vi "Get Control Indexes.vi"(10 "data allocations":T2, 11 "Sequencer Module configuration in":refnum<class "Sequencer Module configuration.lvclass">) -> (0 "error out":errorcluster, 2 "Sequencer Control Index":T1)   [LabVIEW 2015, in "Sequencer Module runtime.lvclass"]
uses:
  Sequencer Module runtime.lvclass
  <vilib>/NI/Tag Bus Module Framework/channel/data tables.ctl
  <vilib>/NI/Tag Bus/dictionary/data dictionary.lvclass
  <vilib>/NI/Tag Bus/dictionary table pair.ctl
  <vilib>/NI/Tag Bus/table/data table.ctl
  configuration/Sequencer Module configuration.lvclass
  Sequencer Control Index.ctl
  <vilib>/NI/Tag Bus Module Framework/channel/TBM channel.lvclass/TBM channel.ctl
  <vilib>/NI/Tag Bus/tag/tag descriptor.lvclass/tag descriptor.ctl
  <vilib>/NI/Tag Bus/tag/read tag name.vi
  <vilib>/NI/Tag Bus/tag/read data type.vi
  <vilib>/NI/Tag Bus/dictionary/locate tag.vi
  <vilib>/NI/Tag Bus Module Framework/channel/TBM channel.lvclass
  <vilib>/NI/Tag Bus/table/data table.lvlib
  <vilib>/NI/Tag Bus/tag bus.lvlib
types:
  T1 = typedef "Sequencer Module runtime.lvclass/Sequencer Control Index.ctl" = cluster{"Start":i32, "Change Sequence":i32, "New Sequence":i32, "Pause":i32}
  T2 = typedef "TBM channel.lvclass/data tables.ctl" = cluster{"input data":T3, "processing parameter":T3, "processing result":T3, "output data":T3}
  T3 = typedef "tag bus.lvlib/dictionary table pair.ctl" = cluster{"data dictionary":refnum<class "data dictionary.lvclass">, "data table":T4}
  T4 = typedef "tag bus.lvlib/data table.lvlib/data table.ctl" = cluster{"Double":dbl[], "Single":sgl[], "I64":i64[], "I32":i32[], "I16":i16[], "I8":i8[], "U64":u64[], "U32":u32[], "U16":u16[], "U8":u8[], "Boolean":bool[], "String":string[], "Array of Double":cluster{"DBL Array":dbl[]}[], "Array of Single":cluster{"SGL Array":sgl[]}[], "Array of I64":cluster{"I64 Array":i64[]}[], "Array of I32":cluster{"I32 Array":i32[]}[], "Array of I16":cluster{"I16 Array":i16[]}[], "Array of I8":cluster{"I8 Array":i8[]}[], "Array of U64":cluster{"U64 Array":u64[]}[], "Array of U32":cluster{"U32 Array":u32[]}[], "Array of U16":cluster{"U16 Array":u16[]}[], "Array of U8":cluster{"U8 Array":u8[]}[], "Array of Boolean":cluster{"Boolean Array":bool[]}[], "Array of String":cluster{"String Array":string[]}[]}
  T5 = typedef "TBM channel.lvclass/channel classification.ctl" = enum16{"input data", "output data", "processing parameter", "processing result"}
  T6 = cluster{"[0]":i32, "[1]":i32, "[2]":i32, "[3]":i32}
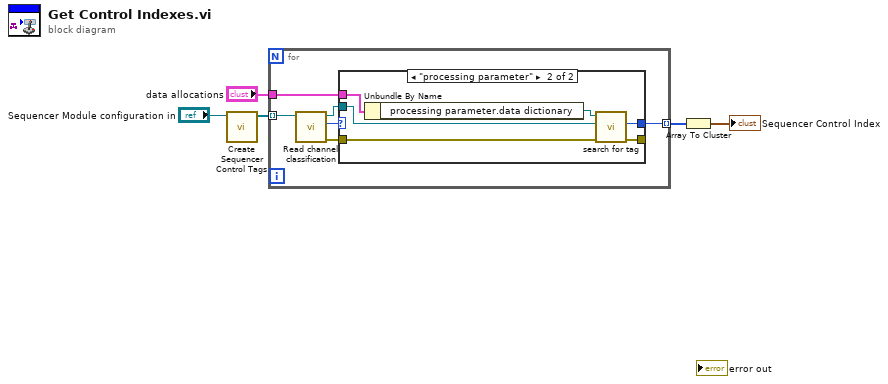
[diagram p0: block diagram]
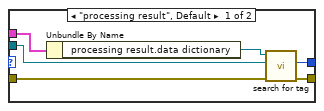
[diagram p2: hidden frame]
diagram:
  n1 = call "Create Sequencer Control Tags.vi"("Sequencer Module configuration in"="Sequencer Module configuration in") -> ("Array"=w1:refnum<class "TBM channel.lvclass">[])  [unwired: 10 in]
  n2 = for {
    tunnel: "data allocations" -> [w8]
    tunnel: w1 -> [w7] mode=indexing
    tunnel: [w6] -> w4 mode=indexing
    n3 = call <vilib>:"Read channel classification.vi"("channel in"=w7) -> ("error out"=w9:errorcluster, "channel classification"=w11:T5, "channel out"=w10:refnum<class "TBM channel.lvclass">)  [unwired: 8 in]
    n4 = case shown="\"processing parameter\"" w11 {
      tunnel: w8 -> [w16 w23]
      tunnel: w10 -> [w12 w21]
      tunnel: [w15 w20] -> w6
      tunnel: w9 -> [w14 w19]
      tunnel: [w13 w18] -> _
      frame "processing result", Default {
        n5 = Unbundle By Name(w16) -> ("processing result.data dictionary"=w17:refnum<class "data dictionary.lvclass">)
        n6 = call <vilib>:"search for tag.vi"("error in"=w14, "system tag"=w12, "data dictionary in"=w17) -> ("error out"=w13:errorcluster, "index"=w15:i32)  [unwired: 6 in, 1 out]
      }
      frame "processing parameter" {
        n7 = Unbundle By Name(w23) -> ("processing parameter.data dictionary"=w22:refnum<class "data dictionary.lvclass">)
        n8 = call <vilib>:"search for tag.vi"("error in"=w19, "system tag"=w21, "data dictionary in"=w22) -> ("error out"=w18:errorcluster, "index"=w20:i32)  [unwired: 6 in, 1 out]
      }
    }
  }
  n9 = Array To Cluster(array=w4) -> (cluster=→"Sequencer Control Index":T6)
